vi "Prepare FDMR plus measurement.vi"(7 "Instr info":T1={"Magnet"={"PSU"="", "T monitor"="", "Last update"=timestamp(0 s since 1904-01-01), "Field [T]"=0.0, "Ramp [mT/s]"=0.0, "Heater"=FALSE, "Ramp state"=enum."At Target"}, "MFLI"={"Lock-in"="", "Multimeter"="", "Last update"=timestamp(0 s since 1904-01-01), "Freq [kHz]"=0.0, "Ampl [mV]"=0.0, "OutEn"=FALSE, "In50 Ohm"=FALSE, "DemEn"=FALSE}, "THz"={"Name"="", "Description"="", "Last update"=timestamp(0 s since 1904-01-01), "Start [GHz]"=0.0, "Im Freq[MHz]"=0.0, "End [GHz]"=0.0}, "VTI"={"TempCtl"="", "Last update"=timestamp(0 s since 1904-01-01), "VTI [K]"=0.0, "Sample [K]"=0.0, "Trap[K]"=0.0, "HePot [K]"=0.0, "Ambient [K]"=0.0}, "Rotator"={"Name"=3, "Last update"=timestamp(0 s since 1904-01-01), "Actuator"=1, "Connected"=FALSE, "Moving"=FALSE, "Target"=FALSE, "Cap [nF]"=0.0, "Position [°]"=0.0}, "Servo"=[], "SMU"={"Name"="", "Last update"=timestamp(0 s since 1904-01-01), "SourFunc"="", "SourValue"=0.0, "MeasFunc"="", "MeasValue"=0.0, "Output"=FALSE}, "PMD"={"Name"="", "Last update"=timestamp(0 s since 1904-01-01), "Position [°]"=0.0, "Speed"=0.0, "Desired [°]"=0.0, "Moving"=FALSE, "reserved"=0.0}, "PwrMonitor"={"Name"="", "Last update"=timestamp(0 s since 1904-01-01), "Outage?"=FALSE, "Low"=FALSE, "No battery"=FALSE, "Battery [%]"=0, "Charging"=FALSE}} {"PwrMonitor"."Last update" format="%<%H:%M:%S>T"; "VTI"."Last update" format="%<%H:%M:%S>T"; "PMD"."Last update" format="%<%H:%M:%S>T"; "SMU"."Last update" format="%<%H:%M:%S>T"; "Servo"."Last update" format="%<%H:%M:%S>T"; "Rotator"."Actuator" items=["Linear", "Roatator", "Goniometer"]; "Rotator"."Name" items=["ANC350res", "ANC350num", "ANC350fps", "Unknown"]; "Rotator"."Last update" format="%<%H:%M:%S>T"; "THz"."Last update" format="%<%H:%M:%S>T"; "MFLI"."Last update" format="%<%H:%M:%S>T"; "Magnet"."Last update" format="%<%H:%M:%S>T"}, 8 "error in (no error)":errorcluster, 9 "Setup":T7={"F_start [GHz]"=0.0, "F_end [GHz]"=0.0, "Field [T]"=0.0, "Points [-]"=0, "Sampling Rate"=15, "ModA [G]"=0.0, "ModF [kHz]"=0.0, "Time const [ms]"=0.0, "Angle [°]"=0.0, "Tmp [K]"=0.0, "Wait [min]"=0.0, "Repeat [-]"=1048576, "Comment"="", "Execute"=FALSE, "Auto-mod"=FALSE} {"Sampling Rate" items=["117 ks/S"=9, "58.6 kS/s"=10, "29.3 kS/s"=11, "14.6 kS/s"=12, "7.32 kS/s"=13, "3.66 kS/s"=14, "1.83 kS/s"=15]; "Time const [ms]" format="%_2e"; "ModF [kHz]" min=0.2 max=120.0; "Repeat [-]" max=1048576; "Tmp [K]" min=-1.0 max=330.0; "Field [T]" min=-16.0 max=16.0}, 10 "VID control":T5 {"Multip" items=["1"=1, "2"=2, "3"=3, "4"=4, "6"=6, "8"=8, "9"=9]; "AMC" items=["9"=9, "12"=12]}, 11 "Referencies in":T6) -> (0 "error out":errorcluster)   [LabVIEW 2024]
uses:
  Datatypes/FDMR+ script line.ctl
  Subsystem modules/Lock-in module/ctl/OSC sampling rate.ctl
  Subsystem modules/Messenger service/Data types/Messenger referencies.ctl
  Datatypes/THz parameters.ctl
  Datatypes/Instr Info.ctl
  Subsystem modules/Magnet module/ctl/RampingOutput.ctl
  Datatypes/Single servo status.ctl
  Subsystem modules/Servo drive module/ctl/Axis names.ctl
  Subsystem modules/Lock-in module/ctl/MFLI_message for module.ctl
  Subsystem modules/Lock-in module/ctl/MFLI_command enum.ctl
  Subsystem modules/Temperature control module/ctl/MSG for VTI.ctl
  Subsystem modules/Temperature control module/ctl/TC commands.ctl
  Subsystem modules/Magnet module/ctl/MSG to magnet.ctl
  Subsystem modules/Magnet module/ctl/Magnet Orders.ctl
  Subsystem modules/Temperature control module/ctl/Set point.ctl
  Subsystem modules/Magnet module/ctl/SetField data.ctl
  Subsystem modules/Magnet module/ctl/Magnet mode public.ctl
  Subsystem modules/Lock-in module/ctl/MFLI_parameter and value.ctl
  Subsystem modules/Lock-in module/ctl/MFLI_node.ctl
  Subsystem modules/Lock-in module/ctl/Mode.ctl
  Subsystem modules/THz module/ctl/THz Message for module.ctl
  Subsystem modules/THz module/ctl/THz commands enum.ctl
  Subsystem modules/THz module/ctl/THz sweep parameters.ctl
  Subsystem modules/Sample rotator/ctl/MSG to Rotator.ctl
  Subsystem modules/Sample rotator/ctl/Rotator commands.ctl
  Subsystem modules/Sample rotator/ctl/Positoin to set.ctl
  Subsystem modules/Lock-in module/Lock-in module.lvlib
  Subsystem modules/Temperature control module/Temperature controller.lvlib
  Subsystem modules/Magnet module/Magnet module.lvlib
  Subsystem modules/THz module/THz source modeule.lvlib
  Subsystem modules/Sample rotator/SampleRotator.lvlib
  Subsystem modules/Messenger service/MessengerLib.lvlib
  Subsystem modules/Servo drive module/Servo drive module.lvlib
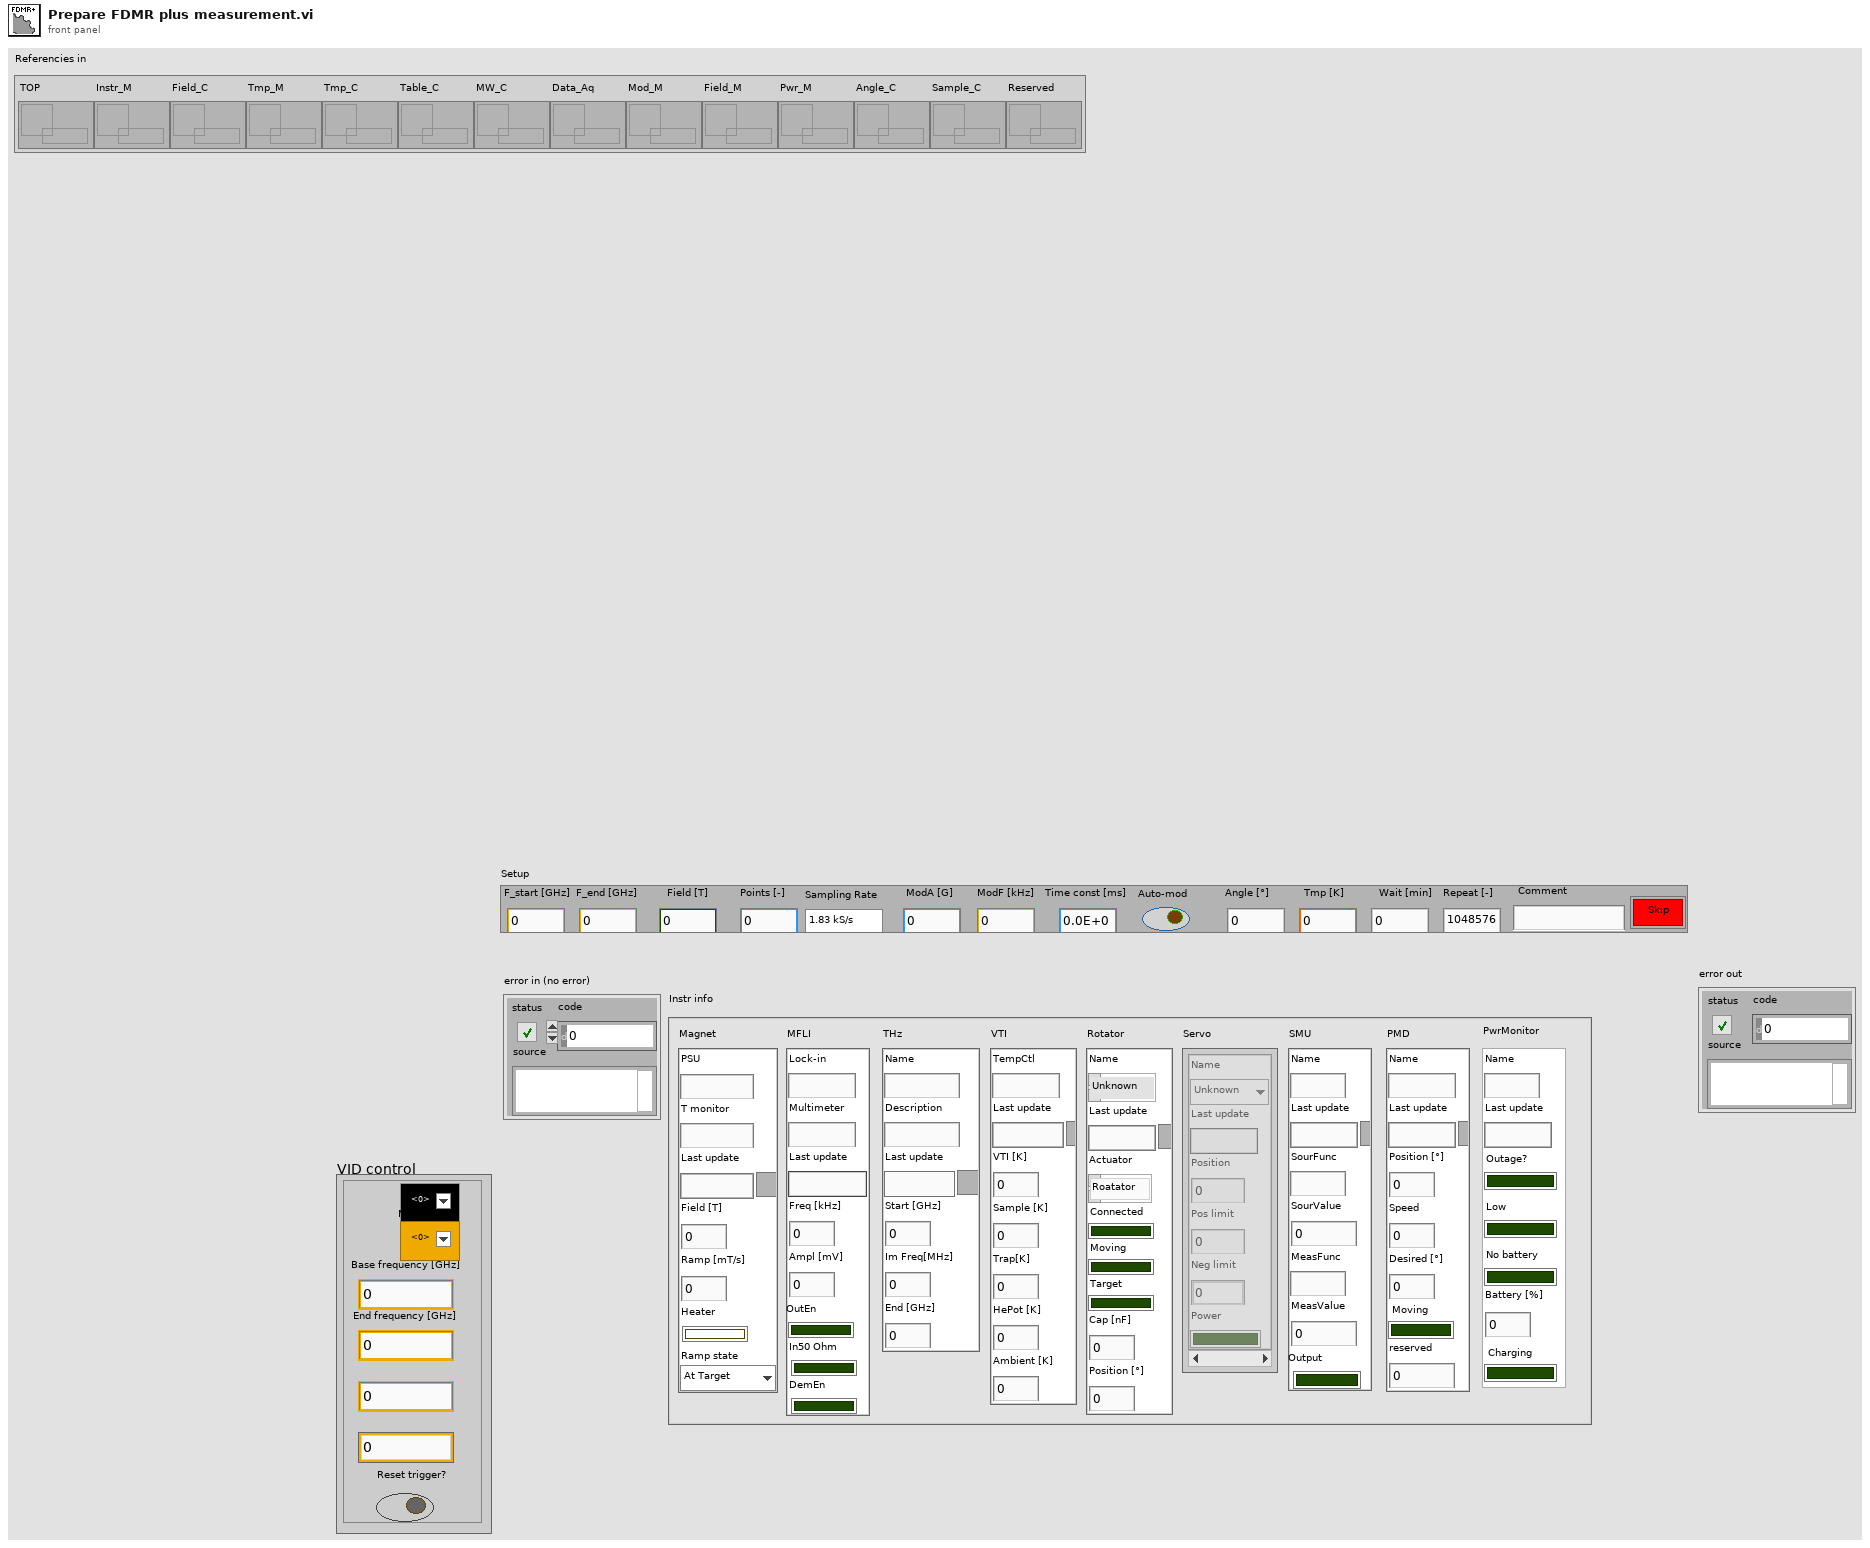
[diagram p1: front panel]
types:
  T1 = typedef "Instr Info.ctl" = cluster{"Magnet":cluster{"PSU":string, "T monitor":string, "Last update":timestamp, "Field [T]":dbl, "Ramp [mT/s]":dbl, "Heater":bool, "Ramp state":T2}, "MFLI":cluster{"Lock-in":string, "Multimeter":string, "Last update":timestamp, "Freq [kHz]":dbl, "Ampl [mV]":dbl, "OutEn":bool, "In50 Ohm":bool, "DemEn":bool}, "THz":cluster{"Name":string, "Description":string, "Last update":timestamp, "Start [GHz]":dbl, "Im Freq[MHz]":dbl, "End [GHz]":dbl}, "VTI":cluster{"TempCtl":string, "Last update":timestamp, "VTI [K]":dbl, "Sample [K]":dbl, "Trap[K]":dbl, "HePot [K]":dbl, "Ambient [K]":dbl}, "Rotator":cluster{"Name":u16, "Last update":timestamp, "Actuator":u16, "Connected":bool, "Moving":bool, "Target":bool, "Cap [nF]":dbl, "Position [°]":dbl}, "Servo":T3[], "SMU":cluster{"Name":string, "Last update":timestamp, "SourFunc":string, "SourValue":dbl, "MeasFunc":string, "MeasValue":dbl, "Output":bool}, "PMD":cluster{"Name":string, "Last update":timestamp, "Position [°]":dbl, "Speed":dbl, "Desired [°]":dbl, "Moving":bool, "reserved":dbl}, "PwrMonitor":cluster{"Name":string, "Last update":timestamp, "Outage?":bool, "Low":bool, "No battery":bool, "Battery [%]":u8, "Charging":bool}}
  T2 = typedef "Magnet module.lvlib/RampingOutput.ctl" = enum16{"At Target", "Go up", "Go down"}
  T3 = typedef "Single servo status.ctl" = cluster{"Name":T4, "Last update":timestamp, "Position":dbl, "Pos limit":dbl, "Neg limit":dbl, "Power":bool}
  T4 = typedef "Servo drive module.lvlib/Axis names.ctl" = enum16{"Unknown", "AxisX", "AxisY", "AxisZ_left", "AxisZ_middle", "AxisZ_right"}
  T5 = typedef "THz parameters.ctl" = cluster{"AMC":u16, "Multip":u16, "Base frequency [GHz]":dbl, "End frequency [GHz]":dbl, "Im frequency [MHz]":dbl, "Sweep up [ms]":dbl, "Reset trigger?":bool}
  T6 = typedef "MessengerLib.lvlib/Messenger referencies.ctl" = cluster{"TOP":refnum<queue>, "Instr_M":refnum<queue>, "Field_C":refnum<queue>, "Tmp_M":refnum<queue>, "Tmp_C":refnum<queue>, "Table_C":refnum<queue>, "MW_C":refnum<queue>, "Data_Aq":refnum<queue>, "Mod_M":refnum<queue>, "Field_M":refnum<queue>, "Pwr_M":refnum<queue>, "Angle_C":refnum<queue>, "Sample_C":refnum<queue>, "Reserved":refnum<queue>}
  T7 = typedef "FDMR+ script line.ctl" = cluster{"F_start [GHz]":dbl, "F_end [GHz]":dbl, "Field [T]":dbl, "Points [-]":u32, "Sampling Rate":T8, "ModA [G]":dbl, "ModF [kHz]":dbl, "Time const [ms]":dbl, "Angle [°]":dbl, "Tmp [K]":dbl, "Wait [min]":dbl, "Repeat [-]":i32, "Comment":string, "Execute":bool, "Auto-mod":bool}
  T8 = typedef "OSC sampling rate.ctl" = u16
  T9 = typedef "Positoin to set.ctl" = cluster{"Relative?":bool, "Position [°]":dbl, "Safe to move?":bool}
  T10 = typedef "SampleRotator.lvlib/MSG to Rotator.ctl" = cluster{"Command":T11, "Data":variant}
  T11 = typedef "SampleRotator.lvlib/Rotator commands.ctl" = enum16{"Ignore", "Initialize", "Update", "Set parameters", "Stop movement", "Set position", "Disconnect", "End"}
  T12 = typedef "Lock-in module.lvlib/MFLI_parameter and value.ctl" = cluster{"parameter":T13, "value":dbl}
  T13 = typedef "Lock-in module.lvlib/MFLI_node.ctl" = enum16{"None", "filter_order [-]", "filter_constant [ms]", "in_diff", "in_autorange", "in_imp50", "in_AC", "osc_freq [kHz]", "out_ampl [V]", "out_autorange", "out_imp50", "enable output", "enamble ampl", "scope_enable", "scope_rate", "scope_len", "scope_trigEn", "AuxOut_amplify", "Phase_deg", "AuxOut_select"}
  T14 = typedef "THz source modeule.lvlib/THz sweep parameters.ctl" = cluster{"Start [GHz]":dbl, "End [GHz] ":dbl, "Sweep up\ntime [ms]":dbl, "Sweep down\ntime [ms]":dbl, "Intermidiate [MHz]":dbl, "Reset trigger":bool}
  T15 = typedef "THz source modeule.lvlib/THz Message for module.ctl" = cluster{"Command":T16, "Data":variant}
  T16 = typedef "THz source modeule.lvlib/THz commands enum.ctl" = enum16{"Ignore", "Connect", "Update", "Set parameters", "Disconnect", "End"}
  T17 = typedef "Lock-in module.lvlib/Mode.ctl" = enum16{"None", "Point", "Scope", "Both", "DAQ"}
  T18 = typedef "Lock-in module.lvlib/MFLI_message for module.ctl" = cluster{"Command":T19, "Data":variant}
  T19 = typedef "Lock-in module.lvlib/MFLI_command enum.ctl" = enum16{"Initialize", "Update", "Set parameters", "Set module", "Set individual parameters", "Get point", "Get array", "Disconnect", "End", "Ignore"}
  T20 = typedef "Magnet module.lvlib/SetField data.ctl" = cluster{"Field [T]":dbl, "Ramp [T/s]":dbl, "Custom Ramp?":bool, "Mode":T21}
  T21 = typedef "Magnet module.lvlib/Magnet mode public.ctl" = enum16{"Persistant", "Ramping"}
  T22 = typedef "Temperature controller.lvlib/Set point.ctl" = cluster{"Heater":string, "Tmp [K]":dbl}
  T23 = typedef "Magnet module.lvlib/MSG to magnet.ctl" = cluster{"Command":T24, "Data":variant}
  T24 = typedef "Magnet module.lvlib/Magnet Orders.ctl" = enum16{"Ignore", "Connect", "Update", "Switch mode", "Set field", "Stop ramping", "Equalize output", "Zero output", "Flip polarity", "Blackout", "Set timer", "Eval temperatures", "Disconnect"}
  T25 = typedef "Temperature controller.lvlib/MSG for VTI.ctl" = cluster{"Command":T26, "Data":variant}
  T26 = typedef "Temperature controller.lvlib/TC commands.ctl" = enum16{"Initialize", "Update", "Stop tmp change", "Set temperature", "Set point", "Disconnect", "End", "Ignore"}
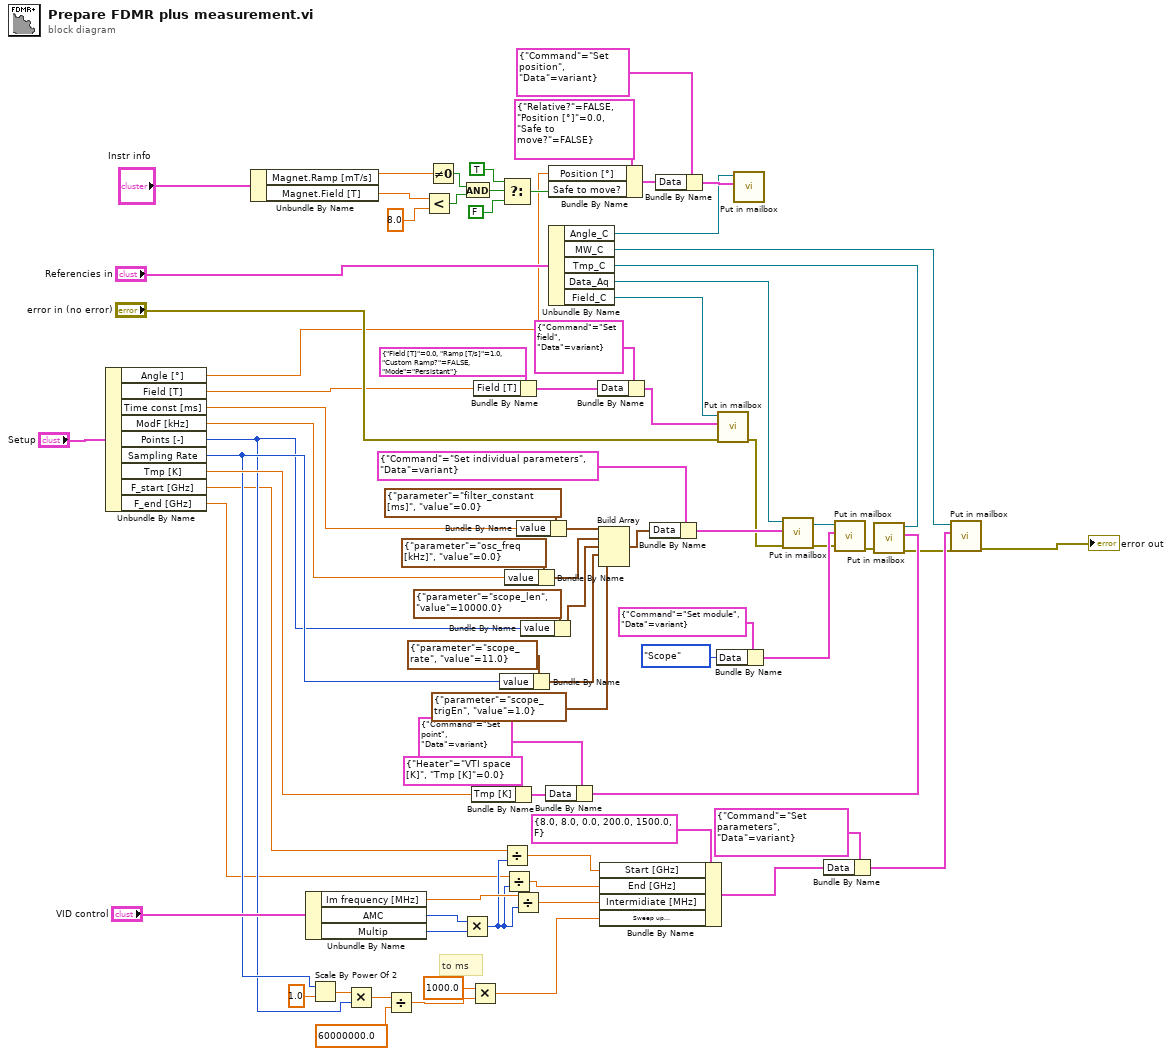
[diagram p0: block diagram]
diagram:
  # "to ms"
  n1 = Unbundle By Name("Setup") -> ("Angle [°]"=w3:dbl, "Field [T]"=w53:dbl, "Time const [ms]"=w61:dbl, "ModF [kHz]"=w60:dbl, "Points [-]"=w23:u32, "Sampling Rate"=w24:T8, "Tmp [K]"=w54:dbl, "F_start [GHz]"=w22:dbl, "F_end [GHz]"=w21:dbl)
  n2 = Unbundle By Name("Instr info") -> ("Magnet.Ramp [mT/s]"=w1:dbl, "Magnet.Field [T]"=w17:dbl)
  n3 = Unbundle By Name("VID control") -> ("Im frequency [MHz]"=w43:dbl, "AMC"=w30:u16, "Multip"=w29:u16)
  n4 = Scale By Power Of 2(n=w24, x=1.0 ("y")) -> (x*2^n=w37:dbl)
  n5 = Multiply(x=w37, y=w23) -> (x*y=w38:dbl)
  n6 = Divide(x=w38, y=60000000.0) -> (x/y=w40:dbl)
  n7 = Less?(x=w17, y=8.0) -> (x < y?=w15:bool)
  n8 = Not Equal To 0?(x=w1) -> (x != 0?=w14:bool)
  n9 = Multiply(x=w30, y=w29) -> (x*y=w28:u16)
  n10 = And(x=w14, y=w15) -> (x .and. y?=w13:bool)
  n11 = Multiply(x=1000.0, y=w40) -> (x*y=w41:dbl)
  n12 = Bundle By Name(cluster=T22 {"Heater"="VTI space [K]", "Tmp [K]"=0.0} ("Set point"), "Tmp [K]"=w54) -> (w70:T22)
  n13 = Bundle By Name(cluster=T20 {"Field [T]"=0.0, "Ramp [T/s]"=1.0, "Custom Ramp?"=FALSE, "Mode"=enum."Persistant"} ("Set Field"), "Field [T]"=w53) -> (w51:T20)
  n14 = Bundle By Name(cluster=T12 {"parameter"=enum."scope_rate", "value"=11.0} ("Parameter to set"), "value"=w24) -> (w56:T12)
  n15 = Select(t=TRUE, s=w13, f=FALSE ("x .and. y?")) -> (s? t:f=w10:bool)
  n16 = Divide(x=w22, y=w28) -> (x/y=w35:dbl)
  n17 = Divide(x=w21, y=w28) -> (x/y=w34:dbl)
  n18 = Bundle By Name(cluster=T12 {"parameter"=enum."osc_freq [kHz]", "value"=0.0} ("Parameter to set"), "value"=w60) -> (w59:T12)
  n19 = Divide(x=w43, y=w28) -> (x/y=w31:dbl)
  n20 = Bundle By Name(cluster=T12 {"parameter"=enum."filter_constant [ms]", "value"=0.0} ("Parameter to set"), "value"=w61) -> (w64:T12)
  n21 = Bundle By Name(cluster=T12 {"parameter"=enum."scope_len", "value"=10000.0} ("Parameter to set"), "value"=w23) -> (w55:T12)
  n22 = Bundle By Name(cluster=T25 {"Command"=enum."Set point", "Data"=variant} ("MSG for VTI"), "Data"=w70) -> (w69:T25)
  n23 = Bundle By Name(cluster=T9 {"Relative?"=FALSE, "Position [°]"=0.0, "Safe to move?"=FALSE} ("Set position"), "Position [°]"=w3, "Safe to move?"=w10) -> (w7:T9)
  n24 = Unbundle By Name("Referencies in") -> ("Angle_C"=w4:refnum<queue>, "MW_C"=w20:refnum<queue>, "Tmp_C"=w79:refnum<queue>, "Data_Aq"=w78:refnum<queue>, "Field_C"=w50:refnum<queue>)
  n25 = Bundle By Name(cluster=T23 {"Command"=enum."Set field", "Data"=variant} ("MSG to magnet"), "Data"=w51) -> (w66:T23)
  n26 = Build Array(w64, w59, w55, w56, T12 {"parameter"=enum."scope_trigEn", "value"=1.0} ("Parameter to set")) -> (w63:T12[])
  n27 = Bundle By Name(cluster=T14 {"Start [GHz]"=8.0, "End [GHz] "=8.0, "Sweep up\ntime [ms]"=0.0, "Sweep down\ntime [ms]"=200.0, "Intermidiate [MHz]"=1500.0, "Reset trigger"=FALSE} ("Sweep parameters"), "Start [GHz]"=w35, "End [GHz]"=w34, "Intermidiate [MHz]"=w31, "Sweep up\ntime [ms]"=w41) -> (w33:T14)
  n28 = Bundle By Name(cluster=T18 {"Command"=enum."Set individual parameters", "Data"=variant} ("MSG for  ACQ"), "Data"=w63) -> (w68:T18)
  n29 = Bundle By Name(cluster=T10 {"Command"=enum."Set position", "Data"=variant} ("MSG to rotator"), "Data"=w7) -> (w8:T10)
  n30 = Bundle By Name(cluster=T18 {"Command"=enum."Set module", "Data"=variant} ("MSG for  ACQ"), "Data"=Mode."Scope" ("Mode")) -> (w48:T18)
  n31 = call "Put in mailbox.vi"("error in (no error)"="error in (no error)", "Message"=w66, "Queue in"=w50) -> ("error out"=w67:errorcluster)  [unwired: 6 in, 2 out]
  n32 = call "Put in mailbox.vi"("Message"=w8, "Queue in"=w4) -> ()  [unwired: 7 in, 3 out]
  n33 = call "Put in mailbox.vi"("error in (no error)"=w67, "Message"=w68, "Queue in"=w78) -> ("error out"=w45:errorcluster, "Queue out"=w46:refnum<queue>)  [unwired: 6 in, 1 out]
  n34 = Bundle By Name(cluster=T15 {"Command"=enum."Set parameters", "Data"=variant} ("Incoming msg"), "Data"=w33) -> (w32:T15)
  n35 = call "Put in mailbox.vi"("error in (no error)"=w45, "Message"=w48, "Queue in"=w46) -> ("error out"=w44:errorcluster)  [unwired: 6 in, 2 out]
  n36 = call "Put in mailbox.vi"("error in (no error)"=w44, "Message"=w69, "Queue in"=w79) -> ("error out"=w19:errorcluster)  [unwired: 6 in, 2 out]
  n37 = call "Put in mailbox.vi"("error in (no error)"=w19, "Message"=w32, "Queue in"=w20) -> ("error out"=→"error out":errorcluster)  [unwired: 6 in, 2 out]
